vi "Main.vi"() -> ()   [LabVIEW 2014]
doc: "This Continuous Measurement sample project is based on the Queued Message Handler template.\n\nThe Event Handling Loop generates messages based on user interface actions.\n\nThe Message Handling Loop processes messages generated by the Event Handling Loop, or by other messages. There are also Acquisition and Logging message handling loop subVIs, and a chart updating loop."
uses:
  Settings/Settings.ctl
  Acquisition/Hardware Configuration.ctl
  Logging/Logging Configuration.ctl
  controls/UI Data.ctl
  controls/UI State.ctl
  support/Message Queue/Enqueue Message (Single).vi
  <vilib>/Utility/error.llb/Error Cluster From Error Code.vi
  <vilib>/ErrorRing/Error Ring.xnode
  Acquisition/Acquisition.lvlib
  Logging/Logging.lvlib
  Settings/Settings.lvlib
  support/User Event - Stop/User Event - Stop.lvlib
  support/Message Queue/Message Queue.lvlib
panel:
  in  "Recording Duration":dbl
  in  "InterRecord Interval":dbl
  out "Data":waveform(dbl)[](graph)
  in  "UserMetaData":T1 {"Amplifier Model" items=["Select a Model", "AM 1700", "BMA 200"]}
  in  "Settings":bool
  in  "Start":bool
  in  "Stop":bool
  out "Status":string
  in  "Exit":bool
  # "Direct-To-Disk Long Term EOD Recording Software (TDMS Output) (1.0)"
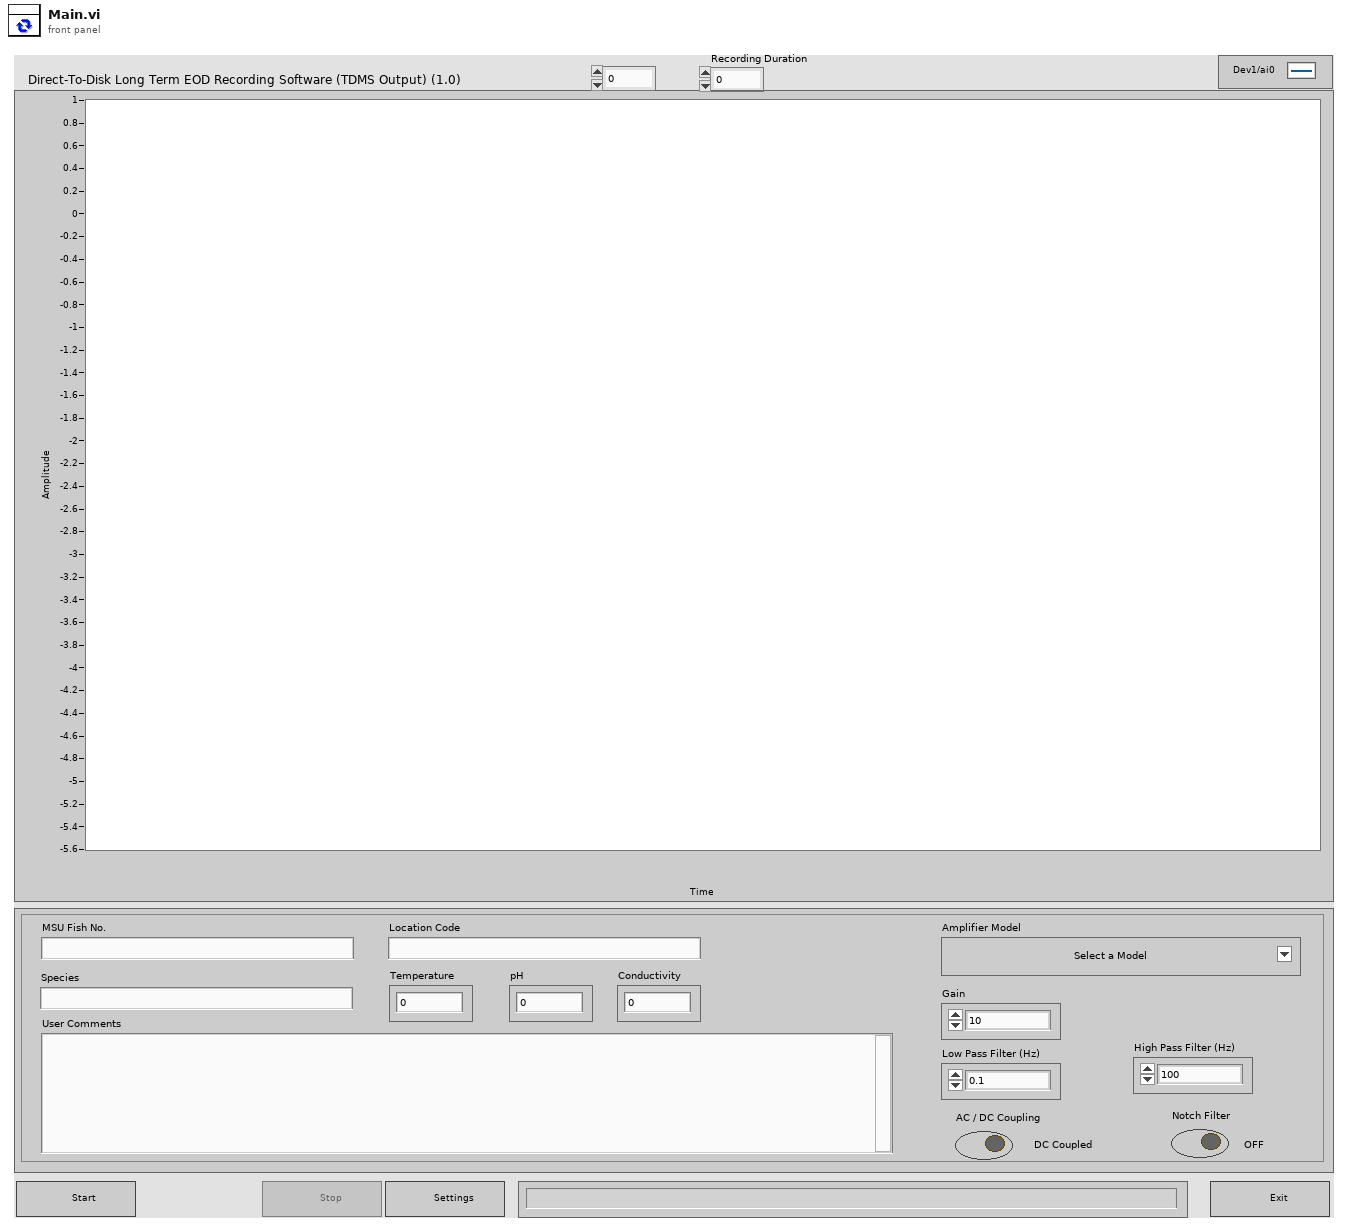
[diagram p1: front panel]
types:
  T1 = cluster{"MSU Fish No.":string, "Location Code":string, "Species":string, "Temperature":dbl, "pH":dbl, "Conductivity":dbl, "User Comments":string, "Amplifier Model":u16, "Gain":enum16{"10", "20", "50", "100", "200", "500", "1000", "2k", "5k", "10k", "20k", "50k"}, "Low Pass Filter (Hz)":enum16{"0.1", "1", "3", "10", "30", "100", "300"}, "High Pass Filter (Hz)":enum16{"100", "500", "1000", "3000", "5000", "10,000", "20,000", "30,000", "50,000"}, "AC / DC Coupling":bool, "Notch Filter":bool}
  T2 = typedef "UI State.ctl" = enum16{"Idle", "Acquiring and Logging", "Waiting for Exit", "Waiting for Exit (Acq Stopped)", "Waiting for Exit (Log Stopped)", "Waiting for Stop", "Waiting for Stop (Acq Stopped)", "Waiting for Stop (Log Stopped)"}
  T3 = typedef "UI Data.ctl" = cluster{"Start Ref":refnum<vi>, "Trigger Ref":refnum<vi>, "Stop Ref":refnum<vi>, "Settings Ref":refnum<vi>, "Status Ref":refnum<vi>, "Exit Ref":refnum<vi>, "Data Ref":refnum<vi>}
  T4 = typedef "Settings.lvlib/Settings.ctl" = cluster{"Hardware Configuration":T5, "Logging Configuration":T6}
  T5 = typedef "Acquisition.lvlib/Hardware Configuration.ctl" = cluster{"DAQmx Channel":tag, "Max Input":dbl, "Min Input":dbl, "Sample Rate":dbl, "DAQmx Task":refnum<k21>}
  T6 = typedef "Logging.lvlib/Logging Configuration.ctl" = cluster{"Log File Base Path":path, "TDMS File Reference":refnum<k34>, "Samples to Save":u32, "Trigger - Time":u32, "Trigger - Threshold":dbl, "Trigger - Channel":u32, "Enable Time Trigger":bool, "Enable Threshold Trigger":bool, "Always Log":bool}
  T7 = typedef "Message Queue.lvlib/All Message Queues.ctl" = cluster{"UI":refnum<queue>, "Acquisition":refnum<queue>, "Logging":refnum<queue>}
  T8 = enum8{"Enabled", "Disabled", "Disabled and Grayed Out"}
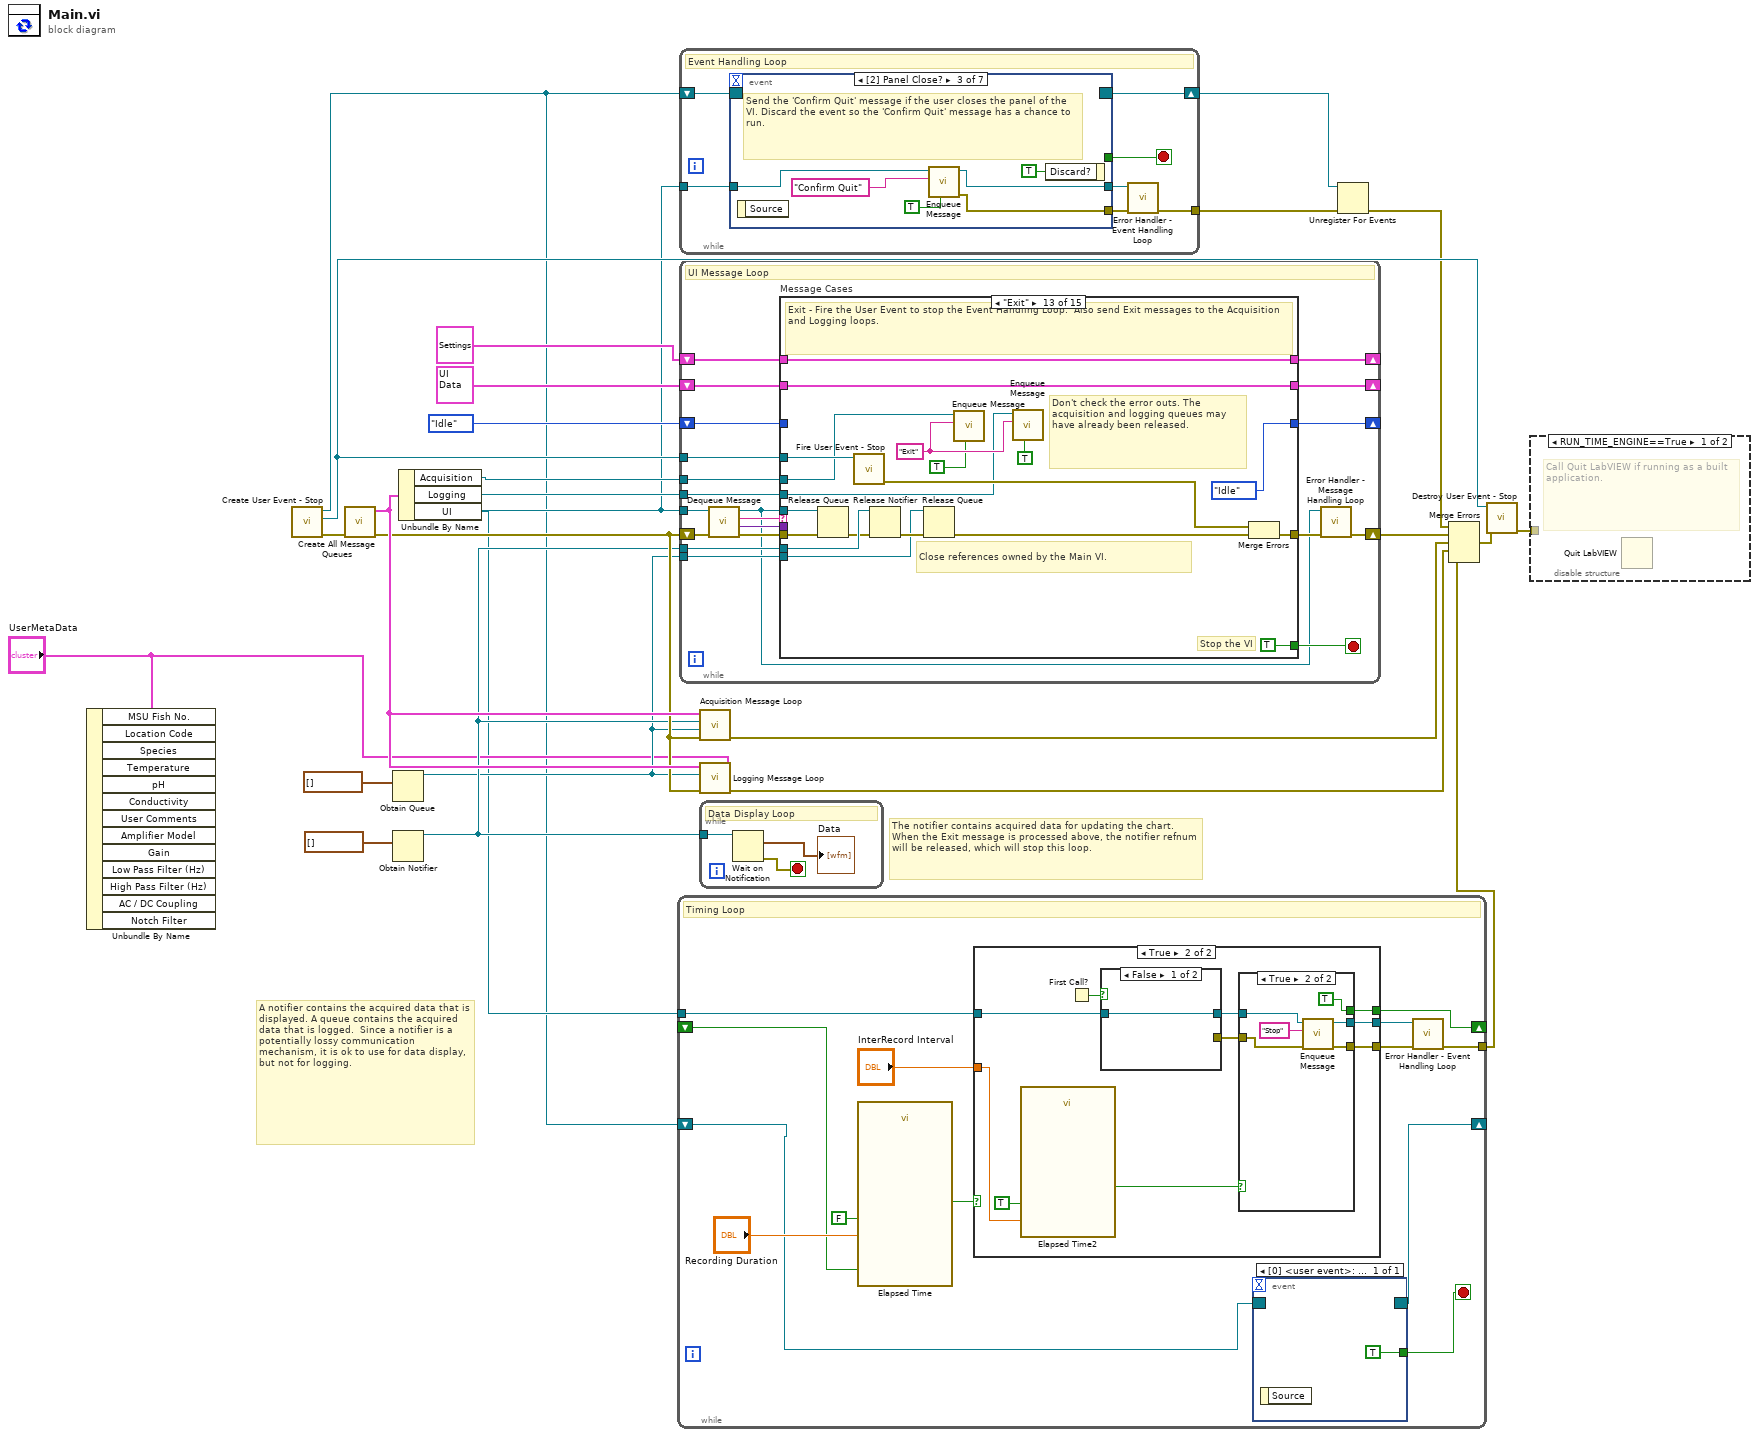
[diagram p0: block diagram]
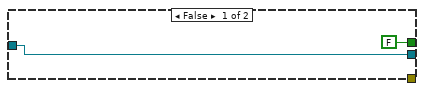
[diagram p2: hidden frame]
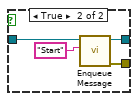
[diagram p3: hidden frame]
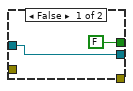
[diagram p4: hidden frame]
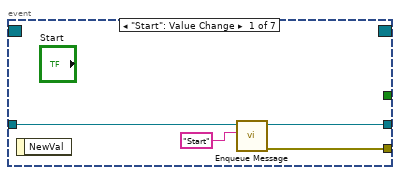
[diagram p6: hidden frame]
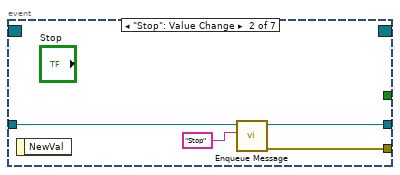
[diagram p7: hidden frame]
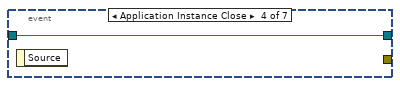
[diagram p8: hidden frame]
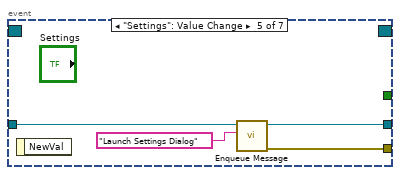
[diagram p9: hidden frame]
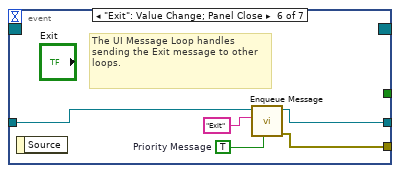
[diagram p10: hidden frame]
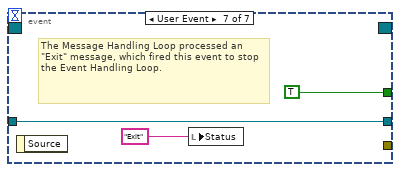
[diagram p11: hidden frame]
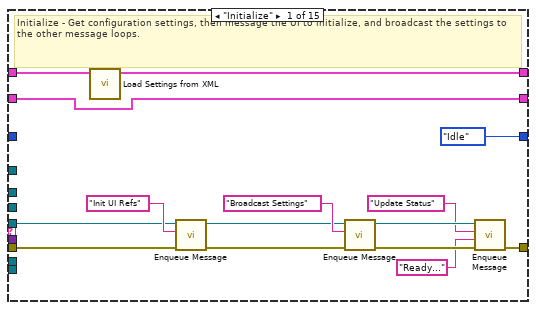
[diagram p12: hidden frame]
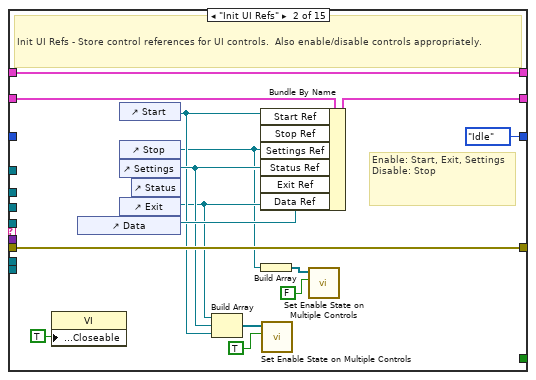
[diagram p13: hidden frame]
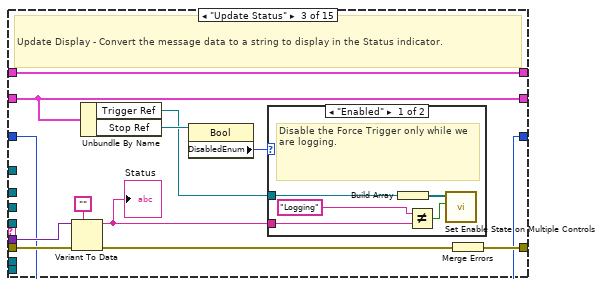
[diagram p14: hidden frame]
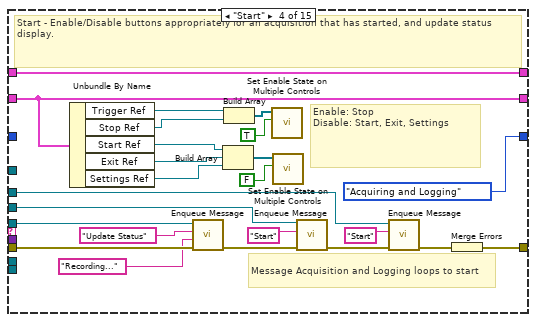
[diagram p16: hidden frame]
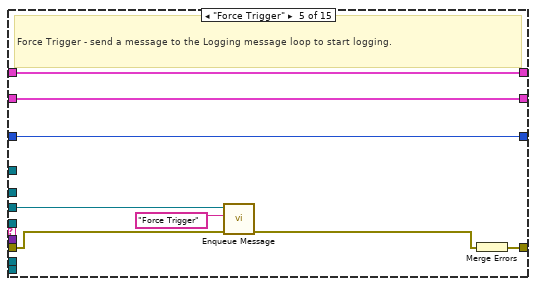
[diagram p17: hidden frame]
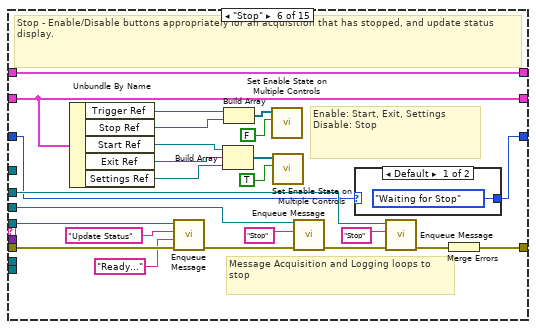
[diagram p18: hidden frame]
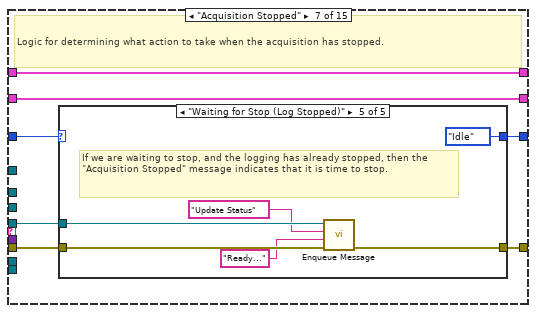
[diagram p20: hidden frame]
diagram:
  # "A notifier contains the acquired data that is displayed. A queue contains the acquired data that is logged.  Since a notifier is a potentially lossy communication mechanism, it is ok to use for data display, but not for logging."
  # "The notifier contains acquired data for updating the chart. When the Exit message is processed above, the notifier refnum will be released, which will stop this loop."
  n1 = Unbundle By Name("UserMetaData") -> ()  [unwired: 13 out]
  n2 = call "Create User Event - Stop.vi"() -> ("error out"=w20:errorcluster, "User Event - Stop"=w22:refnum<user-event>, "Stop Event Registration Refnum"=w1:refnum<event-registration>)  [unwired: 9 in]
  n3 = call "Create All Message Queues.vi"("error in (no error)"=w20) -> ("error out"=w17:errorcluster, "Message Queues out"=w19:T7)  [unwired: 9 in]
  n4 = Obtain Queue(element data type=waveform(dbl)[] []) -> (queue out=w7:refnum<queue>)  [unwired: 4 in, 2 out]
  n5 = Obtain Notifier(notification data type=waveform(dbl)[] []) -> (notifier out=w9:refnum<notifier>)  [unwired: 3 in, 2 out]
  n6 = Unbundle By Name(w19) -> ("Acquisition"=w12:refnum<queue>, "Logging"=w11:refnum<queue>, "UI"=w3:refnum<queue>)
  n7 = while {
    tunnel: w3 -> [w35]
    tunnel: [w36] -> w2
    shift-right: [w30] -> _
    shift-left: _ -> [w29]
    shift-right: [w27] -> _
    shift-left: w1 -> [w28]
    stop <- w26 stop-if-true
    # "Timing Loop"
    n8 = call "Elapsed Time"("Time Target (s)"="Recording Duration", "Reset"=w29, "Auto Reset"=FALSE) -> ("Time has Elapsed"=w37:bool)  [unwired: 9 in, 7 out]
    n9 = case shown="True" w37 {
      tunnel: "InterRecord Interval" -> [_ w50]
      tunnel: w35 -> [w41 w44]
      tunnel: [w41 w48] -> w34
      tunnel: [_ w47] -> w31
      tunnel: [FALSE w46] -> w30
      frame False {
      }
      frame True {
        n10 = call "Elapsed Time2"("Time Target (s)"=w50, "Auto Reset"=TRUE) -> ("Time has Elapsed"=w49:bool)  [unwired: 10 in, 7 out]
        n11 = First Call?() -> (First Call?: T/F=w45:bool)
        n12 = case shown="False" w45 {
          tunnel: [w52 w54] -> w43
          tunnel: w44 -> [w52 w55]
          tunnel: [_ w53] -> w42
          frame False {
          }
          frame True {
            n13 = call-poly "Enqueue Message.vi"("Message"="Start", "Message Queue"=w55) -> ("error out"=w53:errorcluster, "dup Message Queue"=w54:refnum<queue>)  [unwired: 8 in]
          }
        }
        n14 = case shown="True" w49 {
          tunnel: [w57 w64] -> w48
          tunnel: [_ w63] -> w47
          tunnel: [FALSE TRUE] -> w46
          tunnel: w43 -> [w57 w60]
          tunnel: w42 -> [_ w59]
          frame False {
          }
          frame True {
            n15 = call-poly "Enqueue Message.vi"("error in (no error)"=w59, "Message"="Stop", "Message Queue"=w60) -> ("error out"=w63:errorcluster, "dup Message Queue"=w64:refnum<queue>)  [unwired: 7 in]
          }
        }
      }
    }
    n16 = event shown="[0] <user event>: User Event" {
      selector: w28 -> [_]
      dyn-events: [_] -> w27
      timeout: _ -> [_]
      tunnel: [TRUE] -> w26
      event User Event {
        n17 = event-data() -> ()  [unwired: 1 in, 1 out]
      }
    }
    n18 = call "Error Handler - Event Handling Loop.vi"("error in (no error)"=w31, "Message Queue"=w34) -> ("dup error in"=w36:errorcluster)  [unwired: 8 in, 1 out]
  }
  n19 = while {
    tunnel: w3 -> [w70]
    tunnel: [w65] -> w24
    shift-right: [w69] -> w14
    shift-left: w1 -> [w71]
    stop <- w68 stop-if-true
    # "Event Handling Loop"
    n20 = event shown="[2] Panel Close?" {
      selector: w71 -> [_ _ _ _ _ _ _]
      dyn-events: [_ _ _ _ _ _ _] -> w69
      timeout: _ -> [_ _ _ _ _ _ _]
      tunnel: [_ _ _ _ _ _ TRUE ("Discard?")] -> w68
      tunnel: w70 -> [w73 w78 w85 w86 w88 w92 w96]
      tunnel: [w75 w77 w80 _ w90 w95 _] -> w66
      tunnel: [w72 w76 w81 w86 w87 w91 w96] -> w67
      event "Start": Value Change {
        n21 = event-data() -> ()  [unwired: 1 in, 1 out]
        n22 = call-poly "Enqueue Message.vi"("Message"="Start", "Message Queue"=w73) -> ("error out"=w75:errorcluster, "dup Message Queue"=w72:refnum<queue>)  [unwired: 8 in]
      }
      event "Stop": Value Change {
        n23 = event-data() -> ()  [unwired: 1 in, 1 out]
        n24 = call-poly "Enqueue Message.vi"("Message"="Stop", "Message Queue"=w78) -> ("error out"=w77:errorcluster, "dup Message Queue"=w76:refnum<queue>)  [unwired: 8 in]
      }
      event Panel Close? {
        # "Send the 'Confirm Quit' message if the user closes the panel of the VI. Discard the event so the 'Confirm Quit' message has a chance to run."
        n25 = event-data() -> ()  [unwired: 1 in, 1 out]
        n26 = call-poly "Enqueue Message.vi"("Priority Message? (F)"=TRUE, "Message"="Confirm Quit", "Message Queue"=w85) -> ("error out"=w80:errorcluster, "dup Message Queue"=w81:refnum<queue>)  [unwired: 7 in]
        n27 = event-data("Discard?"=TRUE) -> ()  [unwired: 1 in, 1 out]
      }
      event Application Instance Close {
        n28 = event-data() -> ()  [unwired: 1 in, 1 out]
      }
      event "Settings": Value Change {
        n29 = event-data() -> ()  [unwired: 1 in, 1 out]
        n30 = call-poly "Enqueue Message.vi"("Message"="Launch Settings Dialog", "Message Queue"=w88) -> ("error out"=w90:errorcluster, "dup Message Queue"=w87:refnum<queue>)  [unwired: 8 in]
      }
      event "Exit": Value Change; Panel Close {
        w93 = TRUE  # Priority Message
        # "The UI Message Loop handles sending the Exit message to other loops."
        n31 = event-data() -> ()  [unwired: 1 in, 1 out]
        n32 = call-poly "Enqueue Message.vi"("Priority Message? (F)"=w93, "Message"="Exit", "Message Queue"=w92) -> ("error out"=w95:errorcluster, "dup Message Queue"=w91:refnum<queue>)  [unwired: 7 in]
      }
      event User Event {
        # "The Message Handling Loop processed an \"Exit\" message, which fired this event to stop the Event Handling Loop."
        n33 = event-data() -> ()  [unwired: 1 in, 1 out]
        n34 = local write "Status"("Exit" ("Exit String")) -> ()
      }
    }
    n35 = call "Error Handler - Event Handling Loop.vi"("error in (no error)"=w66, "Message Queue"=w67) -> ("dup error in"=w65:errorcluster)  [unwired: 8 in, 1 out]
  }
  n36 = while {
    tunnel: w3 -> [w112]
    tunnel: w22 -> [w117]
    shift-right: [w102] -> w25
    shift-left: w17 -> [w116]
    shift-right: [w111] -> _
    shift-left: T4 {"Hardware Configuration"={"DAQmx Channel"="", "Max Input"=0.0, "Min Input"=0.0, "Sample Rate"=0.0, "DAQmx Task"=""}, "Logging Configuration"={"Log File Base Path"=path "", "TDMS File Reference"=refnum, "Samples to Save"=0, "Trigger - Time"=0, "Trigger - Threshold"=0.0, "Trigger - Channel"=0, "Enable Time Trigger"=FALSE, "Enable Threshold Trigger"=FALSE, "Always Log"=FALSE}} ("Settings") -> [w110]
    shift-right: [w108] -> _
    shift-left: T3 {"Start Ref"=refnum, "Trigger Ref"=refnum, "Stop Ref"=refnum, "Settings Ref"=refnum, "Status Ref"=refnum, "Exit Ref"=refnum, "Data Ref"=refnum} ("Measurement UI Controls") -> [w109]
    tunnel: w12 -> [w107]
    tunnel: w11 -> [w106]
    tunnel: w9 -> [w105]
    tunnel: w7 -> [w104]
    shift-right: [w99] -> _
    shift-left: UI_State."Idle" ("UI State") -> [w100]
    stop <- w118 stop-if-true
    # "UI Message Loop"
    n37 = call "Dequeue Message.vi"("error in (no error)"=w116, "Message Queue"=w112) -> ("error out"=w115:errorcluster, "Message Data"=w113:variant, "Message"=w114:string, "dup Message Queue"=w101:refnum<queue>)  [unwired: 6 in]
    n38 = case "Message Cases" shown="\"Exit\"" w114 {
      selector: w114 -> [_ _ _ _ _ _ _ _ _ _ _ _ _ _ w368]
      tunnel: w101 -> [w123 _ _ w189 _ w222 w226 w251 _ w293 w308 w318 w351 _ _]
      tunnel: w115 -> [w122 w149 w160 w188 w195 w221 w228 w253 w281 w295 w312 w317 w359 w366 _]
      tunnel: [w129 w149 w161 w190 w198 w223 w227 w252 w287 w290 w303 w316 w360 w365 w369] -> w103
      tunnel: [_ _ _ _ _ _ _ _ _ _ _ _ TRUE _ _] -> w118
      tunnel: w113 -> [_ _ w159 _ _ _ _ _ _ _ w311 _ _ _ _]
      tunnel: w117 -> [_ _ _ _ _ _ _ _ _ _ _ _ w358 _ _]
      tunnel: [w132 w148 w156 w187 w197 w220 w232 w257 w285 w292 w314 w321 w356 w364 w371] -> w111
      tunnel: w110 -> [w133 w148 w156 w187 w197 w220 w232 w257 w285 w296 w314 w321 w356 w364 w371]
      tunnel: w109 -> [w125 w147 w155 w184 w196 w217 w231 w256 w279 w289 w313 w320 w354 w363 w370]
      tunnel: [w125 w146 w155 w184 w196 w217 w231 w256 w279 w289 w313 w320 w354 w363 w370] -> w108
      tunnel: w107 -> [_ _ _ w171 _ w204 _ _ w278 _ _ _ w353 _ _]
      tunnel: w106 -> [_ _ _ w174 w192 w207 _ _ w277 _ _ _ w352 _ _]
      tunnel: w105 -> [_ _ _ _ _ _ _ _ _ _ _ _ w350 _ _]
      tunnel: w104 -> [_ _ _ _ _ _ _ _ _ _ _ _ w346 _ _]
      tunnel: w100 -> [_ _ w150 _ w191 w200 w230 w255 w276 w288 w302 w319 _ w362 w367]
      tunnel: [UI_State."Idle" ("UI State") UI_State."Idle" ("UI State") w150 UI_State."Acquiring and Logging" ("UI State") w191 w199 w229 w254 w276 w288 w302 w315 UI_State."Idle" ("UI State") w362 w367] -> w99
      frame "Initialize" {
        # "Initialize - Get configuration settings, then message the UI to initialize, and broadcast the settings to the other message loops."
        n39 = call "Load Settings from XML.vi"("Settings in"=w133) -> ("Settings out"=w132:T4)  [unwired: 9 in, 1 out]
        n40 = call-poly "Enqueue Message.vi"("error in (no error)"=w122, "Message"="Init UI Refs", "Message Queue"=w123) -> ("error out"=w120:errorcluster, "dup Message Queue"=w121:refnum<queue>)  [unwired: 7 in]
        n41 = call-poly "Enqueue Message.vi"("error in (no error)"=w120, "Message"="Broadcast Settings", "Message Queue"=w121) -> ("error out"=w131:errorcluster, "dup Message Queue"=w130:refnum<queue>)  [unwired: 7 in]
        n42 = call-poly "Enqueue Message.vi"("error in (no error)"=w131, "Message Data"="Ready..." ("Ready..."), "Message"="Update Status", "Message Queue"=w130) -> ("error out"=w129:errorcluster)  [unwired: 6 in, 1 out]
      }
      frame "Init UI Refs" {
        # "Enable: Start, Exit, Settings\nDisable: Stop"
        # "Init UI Refs - Store control references for UI controls.  Also enable/disable controls appropriately."
        n43 = property class="VI"("Front Panel.Closeable"=TRUE ("Front Panel Window:Closeable")) -> ()  [unwired: 2 in, 2 out]
        n44 = control-ref of="Data"() -> (w142:refnum<vi>)
        n45 = control-ref of="Start"() -> (w141:refnum<vi>)
        n46 = control-ref of="Stop"() -> (w136:refnum<vi>)
        n47 = control-ref of="Settings"() -> (w138:refnum<vi>)
        n48 = control-ref of="Exit"() -> (w137:refnum<vi>)
        n49 = control-ref of="Status"() -> (w143:refnum<vi>)
        n50 = Build Array(w137, w138, w141) -> (w140:refnum<vi>[])
        n51 = Bundle By Name(cluster=w147, "Start Ref"=w141, "Stop Ref"=w136, "Settings Ref"=w138, "Status Ref"=w143, "Exit Ref"=w137, "Data Ref"=w142) -> (w146:T3)
        n52 = Build Array(w136) -> (w135:refnum<vi>[])
        n53 = call "Set Enable State on Multiple Controls.vi"("Enable?"=TRUE, "Controls"=w140) -> ()  [unwired: 10 in]
        n54 = call "Set Enable State on Multiple Controls.vi"("Enable?"=FALSE, "Controls"=w135) -> ()  [unwired: 10 in]
      }
      frame "Update Status" {
        # "Update Display - Convert the message data to a string to display in the Status indicator."
        n55 = Variant To Data(error in=w160, type="", Variant=w159) -> (data=w152:string, error out=w157:errorcluster)
        "Status" <- w152
        n56 = Unbundle By Name(w155) -> ("Trigger Ref"=w151:refnum<vi>, "Stop Ref"=w154:refnum<vi>)
        n57 = property class="Bool"(reference=w154) -> ("DisabledEnum"=w153:T8)  [unwired: 1 in, 2 out]
        n58 = case shown="\"Enabled\"" w153 {
          tunnel: w152 -> [w164 _]
          tunnel: w151 -> [w165 _]
          frame "Enabled" {
            # "Disable the Force Trigger only while we are logging."
            n59 = Build Array(w165) -> (w166:refnum<vi>[])
            n60 = Not Equal?(x="Logging" ("Logging"), y=w164) -> (x != y?=w162:bool)
            n61 = call "Set Enable State on Multiple Controls.vi"("Enable?"=w162, "Controls"=w166) -> ()  [unwired: 10 in]
          }
          frame "Disabled", Default {
          }
        }
        n62 = Merge Errors(w157) -> (w161:errorcluster)
      }
      frame "Start" {
        # "Message Acquisition and Logging loops to start"
        # "Enable: Stop\nDisable: Start, Exit, Settings"
        # "Start - Enable/Disable buttons appropriately for an acquisition that has started, and update status display."
        n63 = Unbundle By Name(w184) -> ("Trigger Ref"=w168:refnum<vi>, "Stop Ref"=w169:refnum<vi>, "Start Ref"=w179:refnum<vi>, "Exit Ref"=w178:refnum<vi>, "Settings Ref"=w177:refnum<vi>)
        n64 = call-poly "Enqueue Message.vi"("error in (no error)"=w188, "Message Data"="Recording..." ("Waiting for trigger"), "Message"="Update Status", "Message Queue"=w189) -> ("error out"=w176:errorcluster)  [unwired: 6 in, 1 out]
        n65 = Build Array(w179, w178, w177) -> (w182:refnum<vi>[])
        n66 = Build Array(w168, w169) -> (w181:refnum<vi>[])
        n67 = call "Set Enable State on Multiple Controls.vi"("Enable?"=TRUE, "Controls"=w181) -> ()  [unwired: 10 in]
        n68 = call "Set Enable State on Multiple Controls.vi"("Enable?"=FALSE, "Controls"=w182) -> ()  [unwired: 10 in]
        n69 = call-poly "Enqueue Message.vi"("error in (no error)"=w176, "Message"="Start", "Message Queue"=w174) -> ("error out"=w173:errorcluster)  [unwired: 7 in, 1 out]
        n70 = call-poly "Enqueue Message.vi"("error in (no error)"=w173, "Message"="Start", "Message Queue"=w171) -> ("error out"=w172:errorcluster)  [unwired: 7 in, 1 out]
        n71 = Merge Errors(w172) -> (w190:errorcluster)
      }
      frame "Force Trigger" {
        # "Force Trigger - send a message to the Logging message loop to start logging."
        n72 = call-poly "Enqueue Message.vi"("error in (no error)"=w195, "Message"="Force Trigger", "Message Queue"=w192) -> ("error out"=w194:errorcluster)  [unwired: 7 in, 1 out]
        n73 = Merge Errors(w194) -> (w198:errorcluster)
      }
      frame "Stop" {
        # "Message Acquisition and Logging loops to stop"
        # "Enable: Start, Exit, Settings\nDisable: Stop"
        # "Stop - Enable/Disable buttons appropriately for an acquisition that has stopped, and update status display."
        n74 = Unbundle By Name(w217) -> ("Trigger Ref"=w201:refnum<vi>, "Stop Ref"=w202:refnum<vi>, "Start Ref"=w212:refnum<vi>, "Exit Ref"=w211:refnum<vi>, "Settings Ref"=w210:refnum<vi>)
        n75 = call-poly "Enqueue Message.vi"("error in (no error)"=w221, "Message Data"="Ready..." ("Ready..."), "Message"="Update Status", "Message Queue"=w222) -> ("error out"=w209:errorcluster)  [unwired: 6 in, 1 out]
        n76 = Build Array(w212, w211, w210) -> (w215:refnum<vi>[])
        n77 = Build Array(w201, w202) -> (w214:refnum<vi>[])
        n78 = call "Set Enable State on Multiple Controls.vi"("Enable?"=FALSE, "Controls"=w214) -> ()  [unwired: 10 in]
        n79 = call "Set Enable State on Multiple Controls.vi"("Enable?"=TRUE, "Controls"=w215) -> ()  [unwired: 10 in]
        n80 = call-poly "Enqueue Message.vi"("error in (no error)"=w209, "Message"="Stop", "Message Queue"=w207) -> ("error out"=w206:errorcluster)  [unwired: 7 in, 1 out]
        n81 = case shown="Default" w200 {
          selector: w200 -> [_ w225]
          tunnel: [UI_State."Waiting for Stop" ("UI State") w225] -> w199
          frame Default {
          }
          frame "Waiting for Exit" {
          }
        }
        n82 = call-poly "Enqueue Message.vi"("error in (no error)"=w206, "Message"="Stop", "Message Queue"=w204) -> ("error out"=w205:errorcluster)  [unwired: 7 in, 1 out]
        n83 = Merge Errors(w205) -> (w223:errorcluster)
      }
      frame "Acquisition Stopped" {
        # "Logic for determining what action to take when the acquisition has stopped."
        n84 = case shown="\"Waiting for Stop (Log Stopped)\"" w230 {
          selector: w230 -> [w234 _ _ _ _]
          tunnel: [w234 UI_State."Waiting for Exit (Acq Stopped)" ("UI State") UI_State."Waiting for Stop (Acq Stopped)" ("UI State") UI_State."Idle" ("UI State") UI_State."Idle" ("UI State")] -> w229
          tunnel: w228 -> [w233 w235 w237 w243 w249]
          tunnel: [w233 w235 w237 w242 w248] -> w227
          tunnel: w226 -> [_ _ _ w241 w247]
          frame Default {
          }
          frame "Waiting for Exit", "Waiting for Exit (Acq Stopped)" {
          }
          frame "Waiting for Stop", "Waiting for Stop (Acq Stopped)" {
          }
          frame "Waiting for Exit (Log Stopped)" {
            # "If we are waiting to exit, and the logging has already stopped, then the \"Acquisition Stopped\" message indicates that it is time to exit."
            n85 = call-poly "Enqueue Message.vi"("Priority Message? (F)"=TRUE, "error in (no error)"=w243, "Message"="Exit", "Message Queue"=w241) -> ("error out"=w242:errorcluster)  [unwired: 6 in, 1 out]
          }
          frame "Waiting for Stop (Log Stopped)" {
            # "If we are waiting to stop, and the logging has already stopped, then the \"Acquisition Stopped\" message indicates that it is time to stop."
            n86 = call-poly "Enqueue Message.vi"("error in (no error)"=w249, "Message Data"="Ready..." ("Message"), "Message"="Update Status", "Message Queue"=w247) -> ("error out"=w248:errorcluster)  [unwired: 6 in, 1 out]
          }
        }
      }
      frame "Logging Stopped" {
        # "Logic for determining what action to take when the logging has stopped."
        n87 = case shown="\"Waiting for Stop (Acq Stopped)\"" w255 {
          selector: w255 -> [w259 _ _ _ _]
          tunnel: [w259 UI_State."Waiting for Exit (Log Stopped)" ("UI State") UI_State."Waiting for Stop (Log Stopped)" ("UI State") UI_State."Idle" ("UI State") UI_State."Idle" ("UI State")] -> w254
          tunnel: w253 -> [w258 w260 w262 w268 w274]
          tunnel: [w258 w260 w262 w267 w273] -> w252
          tunnel: w251 -> [_ _ _ w266 w272]
          frame Default {
          }
          frame "Waiting for Exit", "Waiting for Exit (Log Stopped)" {
          }
          frame "Waiting for Stop", "Waiting for Stop (Log Stopped)" {
          }
          frame "Waiting for Exit (Acq Stopped)" {
            # "If we are waiting to exit, and the acquisition has already stopped, then the \"Logging Stopped\" message indicates that it is time to exit."
            n88 = call-poly "Enqueue Message.vi"("Priority Message? (F)"=TRUE, "error in (no error)"=w268, "Message"="Exit", "Message Queue"=w266) -> ("error out"=w267:errorcluster)  [unwired: 6 in, 1 out]
          }
          frame "Waiting for Stop (Acq Stopped)" {
            # "If we are waiting to stop, and the acquisition has already stopped, then the \"Logging Stopped\" message indicates that it is time to stop."
            n89 = call-poly "Enqueue Message.vi"("error in (no error)"=w274, "Message Data"="Ready..." ("Message"), "Message"="Update Status", "Message Queue"=w272) -> ("error out"=w273:errorcluster)  [unwired: 6 in, 1 out]
          }
        }
      }
      frame "Broadcast settings" {
        w280 = "Update Settings" ("Message")
        # "Send the 'Update Settings' message to the Logging and Acquisition message loops."
        n90 = Unbundle By Name(w285) -> ("Hardware Configuration"=w284:T5, "Logging Configuration"=w283:T6)
        n91 = call-poly "Enqueue Message.vi"("Message Data"=w284, "Message"=w280, "Message Queue"=w278) -> ("error out"=w286:errorcluster)  [unwired: 7 in, 1 out]
        n92 = call-poly "Enqueue Message.vi"("error in (no error)"=w286, "Message Data"=w283, "Message"=w280, "Message Queue"=w277) -> ("error out"=w282:errorcluster)  [unwired: 6 in, 1 out]
        n93 = Merge Errors(w282, w281) -> (w287:errorcluster)
      }
      frame "Launch Settings Dialog" {
        # "Launch the Settings Dialog when the user clicks the 'Settings' button."
        n94 = call "Settings Dialog.vi"("error in (no error)"=w295, "Settings in"=w296) -> ("error out"=w291:errorcluster, "Cancelled?"=w294:bool, "Settings out"=w292:T4)  [unwired: 6 in, 1 out]
        n95 = case shown="False" w294 {
          tunnel: w293 -> [w300 _]
          tunnel: w291 -> [w299 w301]
          tunnel: [w298 w301] -> w290
          frame False {
            n96 = call-poly "Enqueue Message.vi"("error in (no error)"=w299, "Message"="Broadcast Settings", "Message Queue"=w300) -> ("error out"=w298:errorcluster)  [unwired: 7 in, 1 out]
          }
          frame True {
          }
        }
      }
      frame "Error" {
        # "Error - Check the error message data and respond accordingly. This message is sent by the \"Error Handler\" VIs at the end of each loop in this application."
        n97 = Variant To Data(error in=w312, type=errorcluster {"status"=FALSE, "code"=0, "source"=""} ("error out"), Variant=w311) -> (data=w309:errorcluster, error out=w305:errorcluster)
        n98 = call <vilib>:"Simple Error Handler.vi"("error in (no error)"=w309) -> ()  [unwired: 4 in, 5 out]
        n99 = call-poly "Enqueue Message.vi"("Priority Message? (F)"=TRUE, "Message"="Exit", "Message Queue"=w308) -> ("error out"=w304:errorcluster)  [unwired: 7 in, 1 out]
        n100 = Merge Errors(w304, w305) -> (w303:errorcluster)
      }
      frame "Confirm Quit" {
        # "Confirm Quit - Message that can confirm whether or not the user wants to exit the application."
        n101 = case shown="\"Acquiring and Logging\"" w319 {
          tunnel: w318 -> [w326 w332]
          tunnel: w317 -> [w325 w330]
          tunnel: [w322 w329] -> w316
          tunnel: [UI_State."Idle" ("UI State") w328] -> w315
          frame Default {
            # "If 'Confirm Quit' comes in while the system is idle, there is no need for a confirmation message."
            n102 = call-poly "Enqueue Message.vi"("Priority Message? (F)"=TRUE, "error in (no error)"=w325, "Message"="Exit", "Message Queue"=w326) -> ("error out"=w322:errorcluster)  [unwired: 6 in, 1 out]
          }
          frame "Acquiring and Logging" {
            n103 = Two Button Dialog(message="Are you sure you want to quit while the acquisition is running?" ("Confirm Quit Message"), 1:"No" ("No"), 2:"Yes" ("Yes")) -> (T button?=w331:bool)
            n104 = case shown="True" w331 {
              tunnel: w332 -> [_ w342]
              tunnel: w330 -> [w336 w341]
              tunnel: [w336 w340] -> w329
              tunnel: [UI_State."Acquiring and Logging" ("UI State") UI_State."Waiting for Exit" ("UI State")] -> w328
              frame False {
                # "User did not want to quit."
              }
              frame True {
                n105 = call-poly "Enqueue Message.vi"("error in (no error)"=w341, "Message"="Stop", "Message Queue"=w342) -> ("error out"=w340:errorcluster)  [unwired: 7 in, 1 out]
              }
            }
          }
        }
      }
      frame "Exit" {
        w355 = "Exit" ("Message")
        # "Don't check the error outs. The acquisition and logging queues may have already been released."
        # "Close references owned by the Main VI."
        # "Stop the VI"
        # "Exit - Fire the User Event to stop the Event Handling Loop.  Also send Exit messages to the Acquisition and Logging loops."
        n106 = Release Queue(queue=w351, error in (no error)=w359) -> (error out=w349:errorcluster)  [unwired: 1 in, 2 out]
        n107 = call "Fire User Event - Stop.vi"("User Event - Stop"=w358) -> ("error out"=w357:errorcluster)  [unwired: 10 in]
        n108 = Release Notifier(notifier=w350, error in (no error)=w349) -> (error out=w348:errorcluster)  [unwired: 1 in, 2 out]
        n109 = Release Queue(queue=w346, error in (no error)=w348) -> (error out=w347:errorcluster)  [unwired: 1 in, 2 out]
        n110 = call-poly "Enqueue Message.vi"("Priority Message? (F)"=TRUE, "Message"=w355, "Message Queue"=w353) -> ()  [unwired: 7 in, 2 out]
        n111 = call-poly "Enqueue Message.vi"("Priority Message? (F)"=TRUE, "Message"=w355, "Message Queue"=w352) -> ()  [unwired: 7 in, 2 out]
        n112 = Merge Errors(w357, w347) -> (w360:errorcluster)
      }
      frame "---Copy This Frame---" {
        # "Duplicate this frame when creating new messages.  Change this comment in the duplicated frame to describe this message."
        n113 = Merge Errors(w366) -> (w365:errorcluster)
      }
      frame Default {
        # "'Default' case only runs if there is a message that isn't defined in any of the other cases.  Output a programming error."
        n114 = xnode "Error Ring"("parameter 0"=w368) -> ("error out"=w369:errorcluster)
      }
    }
    n115 = call "Error Handler - Message Handling Loop.vi"("error in (no error)"=w103, "Message Queue"=w101) -> ("dup error in"=w102:errorcluster)  [unwired: 8 in, 1 out]
  }
  n116 = call "Acquisition Message Loop.vi"("error in (no error)"=w17, "Data Queue"=w7, "Data Notifier"=w9, "Message Queues"=w19) -> ("error out"=w21:errorcluster)  [unwired: 7 in]
  n117 = call "Logging Message Loop.vi"("UserMetaData"="UserMetaData", "error in (no error)"=w17, "Data Queue"=w7, "Message Queues"=w19) -> ("error out"=w18:errorcluster)  [unwired: 7 in]
  n118 = while "Data Display Loop" {
    tunnel: w9 -> [w381]
    stop <- w379 stop-if-true
    # "Data Display Loop"
    n119 = Wait on Notification(notifier=w381) -> (notification=→"Data":waveform(dbl)[], error out=w379:errorcluster)  [unwired: 3 in, 2 out]
  }
  n120 = Unregister For Events(event registration refnum=w14, error in=w24) -> (error out=w15:errorcluster)
  n121 = Merge Errors(w15, w25, w21, w18, w2) -> (w23:errorcluster)
  n122 = call "Destroy User Event - Stop.vi"("error in (no error)"=w23, "User Event - Stop"=w22) -> ("error out"=w6:errorcluster)  [unwired: 9 in]
  n123 = disable-structure shown="RUN_TIME_ENGINE==True" {
    disable-tunnel: w6 -> [_ _]
    frame condition #0 {
      # "Call Quit LabVIEW if running as a built application."
      n124 = Quit LabVIEW() -> ()  [unwired: 1 in]
    }
    frame condition #1 (active) {
    }
  }
